vi "API - Update Tx Packet Order.vi"(6 "Channel Names":string[](array[string]), 8 "error in (no error)":errorcluster, 11 "Node Ptr":T1 format="%.0x") -> (0 "error out":errorcluster, 3 "Node Ptr out":T1 format="%.0x")   [LabVIEW 2016, in "UDP-Custom-Device System Explorer.lvlib"]
uses:
  UDP-Custom-Device System Explorer.lvlib
  <vilib>/NI Veristand/Custom Device API/Custom Device Item Ref.ctl
  Shared/Constants.vi
  <vilib>/NI Veristand/Custom Device API/Set Item Property (I32).vi
  <vilib>/NI VeriStand/Custom Device API/Custom Device API.lvlib
  <vilib>/NI VeriStand/Custom Device Tools/Custom Device Utility Library/Custom Device Utility Library.lvlib
  Shared/UDP-Custom-Device Shared.lvlib
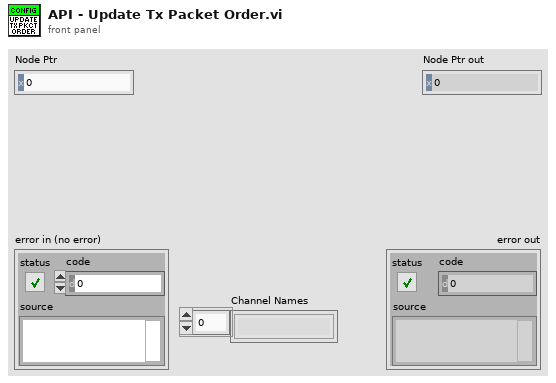
[diagram p1: front panel]
types:
  T1 = typedef "Custom Device API.lvlib/Custom Device Item Ref.ctl" = u64
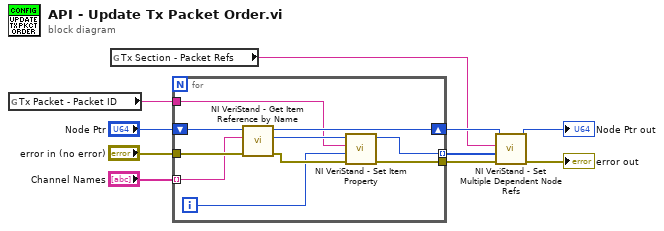
[diagram p0: block diagram]
diagram:
  n1 = global read "Constants.vi" "Tx Packet - Packet ID"() -> (w1:string)
  n2 = global read "Constants.vi" "Tx Section - Packet Refs"() -> (w5:string)
  n3 = for {
    tunnel: "error in (no error)" -> [w20]
    tunnel: "Channel Names" -> [w18] mode=indexing
    shift-right: [w17] -> w7
    shift-left: "Node Ptr" -> [w19]
    tunnel: [w13] -> w6 mode=indexing
    tunnel: [w15] -> w4
    tunnel: w1 -> [w11]
    i -> [w12]
    n4 = call <vilib>:"NI VeriStand - Get Item Reference by Name.vi"("error in (no error)"=w20, "Item Name"=w18, "Parent Ref in"=w19) -> ("error out"=w16:errorcluster, "Item Ref"=w14:T1, "Parent Ref out"=w17:T1)  [unwired: 5 in, 1 out]
    n5 = call-poly <vilib>:"NI VeriStand - Set Item Property.vi"("error in (no error)"=w16, "Value"=w12, "Property Name"=w11, "Item Ref in"=w14) -> ("error out"=w15:errorcluster, "Item Ref out"=w13:T1)  [unwired: 5 in, 1 out]
  }
  n6 = call <vilib>:"NI VeriStand - Set Multiple Dependent Node Refs.vi"("error in (no error)"=w4, "Dependent Node Refs"=w6, "Base Property Name"=w5, "Item Ref in"=w7) -> ("error out"=→"error out":errorcluster, "Item Ref out"=→"Node Ptr out":T1)  [unwired: 6 in]
